vi "ncx_szof.vi"(1 "nc_type":T1(ring)) -> (0 "sz":u64)   [LabVIEW 2016]
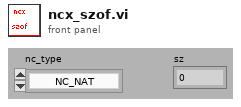
[diagram p1: front panel]
types:
  T1 = enum16{"NC_NAT", "NC_BYTE", "NC_CHAR", "NC_SHORT", "NC_INT", "NC_FLOAT", "NC_DOUBLE"}
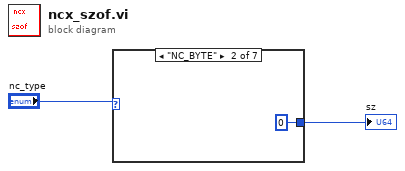
[diagram p0: block diagram]
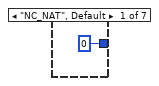
[diagram p2: hidden frame]
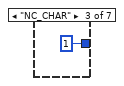
[diagram p3: hidden frame]
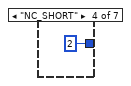
[diagram p4: hidden frame]
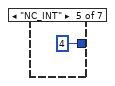
[diagram p5: hidden frame]
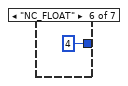
[diagram p6: hidden frame]
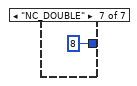
[diagram p7: hidden frame]
diagram:
  n1 = case shown="\"NC_BYTE\"" "nc_type" {
    tunnel: [u64 0 u64 0 u64 1 u64 2 u64 4 u64 4 u64 8] -> w2
    frame "NC_NAT", Default {
    }
    frame "NC_BYTE" {
    }
    frame "NC_CHAR" {
    }
    frame "NC_SHORT" {
    }
    frame "NC_INT" {
    }
    frame "NC_FLOAT" {
    }
    frame "NC_DOUBLE" {
    }
  }
  "sz" <- w2
